vi "Set AI Node Value.vi"(9 "Value":T1, 10 "Location":i32, 11 "Board State In":i32) -> (3 "Board State Out":i32)   [LabVIEW 2013]
uses:
  Typedef/Cell.ctl
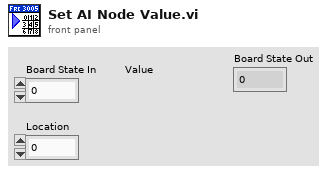
[diagram p1: front panel]
types:
  T1 = typedef "Cell.ctl" = enum16{"", "X", "O"}
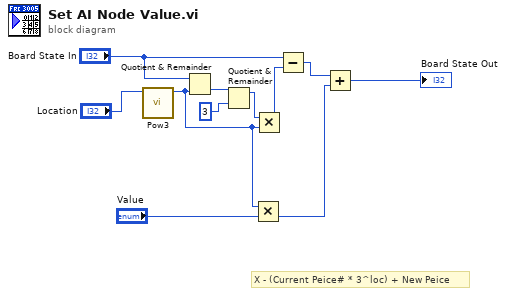
[diagram p0: block diagram]
diagram:
  # "X - (Current Peice# * 3^loc) + New Peice"
  n1 = call "Pow3.vi"("x"="Location") -> ("x^3"=w5:i32)  [unwired: 10 in]
  n2 = Quotient & Remainder(x="Board State In", y=w5) -> (floor(x/y)=w3:i32)  [unwired: 1 out]
  n3 = Quotient & Remainder(x=w3, y=3) -> (x-y*floor(x/y)=w1:i32)  [unwired: 1 out]
  n4 = Multiply(x=w5, y="Value") -> (x*y=w6:i32)
  n5 = Multiply(x=w1, y=w5) -> (x*y=w9:i32)
  n6 = Subtract(x="Board State In", y=w9) -> (x-y=w8:i32)
  n7 = Add(x=w8, y=w6) -> (x+y=→"Board State Out":i32)
